vi "Register gRPC Methods.vi"(8 "error in (no error)":errorcluster, 11 "Template Server in":refnum<class "ctet_dio.lvclass">) -> (0 "error out":errorcluster, 3 "Template Server out":refnum<class "ctet_dio.lvclass">)   [LabVIEW 2019, in "ctet_dio.lvlib" / "ctet_dio.lvclass"]
uses:
  ctet_dio.lvclass
  typeDefs/Server Internal UEs.ctl
  typeDefs/Server Internal Message.ctl
  typeDefs/Server gRPC UEs.ctl
  gRPC lvSupport/Server API/typeDefs/gRPCId Cluster.ctl
  gRPC lvSupport/Server API/typeDefs/grpcId.ctl
  ctet_dio.lvclass/ctet_dio.ctl
  gRPC lvSupport/gprc-lvsupport.lvlib
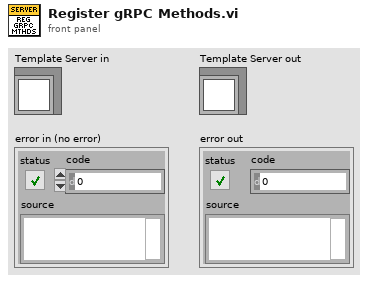
[diagram p1: front panel]
types:
  T1 = typedef "ctet_dio.lvlib/ctet_dio.lvclass/Server gRPC UEs.ctl" = cluster{"Invoke gRPC UE":refnum<user-event>, "Query gRPC UE":refnum<user-event>, "Register gRPC UE":refnum<user-event>, "OpenDISession gRPC UE":refnum<user-event>, "OpenDOSession gRPC UE":refnum<user-event>, "ReadDI gRPC UE":refnum<user-event>, "StopDI gRPC UE":refnum<user-event>, "WriteDO gRPC UE":refnum<user-event>, "CloseDISession gRPC UE":refnum<user-event>, "CloseDOSession gRPC UE":refnum<user-event>}
  T2 = typedef "ctet_dio.lvlib/ctet_dio.lvclass/Server Internal UEs.ctl" = cluster{"Invoke Internal UE":refnum<user-event>, "Query Internal UE":refnum<user-event>, "Register Internal UE":refnum<user-event>, "OpenDISession Internal UE":refnum<user-event>, "OpenDOSession Internal UE":refnum<user-event>, "ReadDI Internal UE":refnum<user-event>, "StopDI Internal UE":refnum<user-event>, "WriteDO Internal UE":refnum<user-event>, "CloseDISession Internal UE":refnum<user-event>, "CloseDOSession Internal UE":refnum<user-event>}
  T3 = typedef "ctet_dio.lvlib/gprc-lvsupport.lvlib/grpcId.ctl" = u64
  T4 = typedef "ctet_dio.lvlib/ctet_dio.lvclass/Server Internal Message UE.ctl" = refnum<user-event>
  T5 = typedef "ctet_dio.lvlib/gprc-lvsupport.lvlib/gRPCId Cluster UE.ctl" = refnum<user-event>
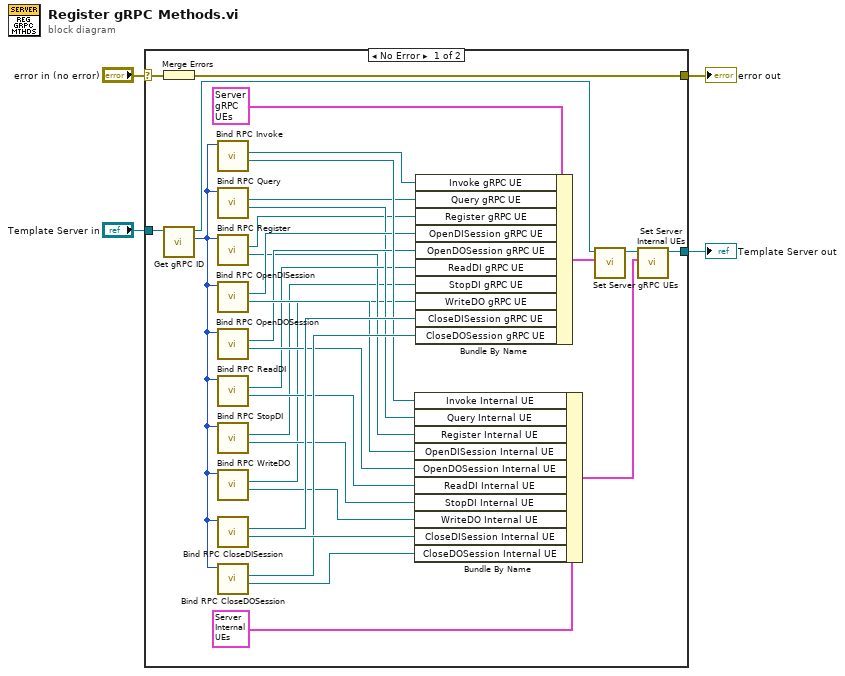
[diagram p0: block diagram]
diagram:
  n1 = case shown="No Error" "error in (no error)" {
    selector: "error in (no error)" -> [w26 w36]
    tunnel: "Template Server in" -> [w34 w37]
    tunnel: [w33 w36] -> w3
    tunnel: [w32 w37] -> w2
    frame No Error {
      n2 = Merge Errors(w26) -> (w33:errorcluster)
      n3 = call "Get gRPC ID.vi"("OOP Server in"=w34) -> ("gRPC ID"=w25:T3, "OOP Server out"=w35:refnum<class "ctet_dio.lvclass">)  [unwired: 9 in]
      n4 = call "Bind RPC Invoke.vi"("gRPCid server in"=w25) -> ("Invoke Internal UE"=w20:T4, "Invoke gRPC UE"=w19:T5)  [unwired: 7 in, 2 out]
      n5 = call "Bind RPC Query.vi"("gRPCid server in"=w25) -> ("Query Internal UE"=w14:T4, "Query gRPC UE"=w13:T5)  [unwired: 7 in, 2 out]
      n6 = call "Bind RPC Register.vi"("gRPCid server in"=w25) -> ("Register Internal UE"=w10:T4, "Register gRPC UE"=w9:T5)  [unwired: 7 in, 2 out]
      n7 = call "Bind RPC OpenDISession.vi"("gRPCid server in"=w25) -> ("OpenDISession Internal UE"=w18:T4, "OpenDISession gRPC UE"=w17:T5)  [unwired: 7 in, 2 out]
      n8 = call "Bind RPC OpenDOSession.vi"("gRPCid server in"=w25) -> ("OpenDOSession Internal UE"=w16:T4, "OpenDOSession gRPC UE"=w15:T5)  [unwired: 7 in, 2 out]
      n9 = call "Bind RPC ReadDI.vi"("gRPCid server in"=w25) -> ("ReadDI Internal UE"=w12:T4, "ReadDI gRPC UE"=w11:T5)  [unwired: 7 in, 2 out]
      n10 = call "Bind RPC StopDI.vi"("gRPCid server in"=w25) -> ("StopDI Internal UE"=w8:T4, "StopDI gRPC UE"=w7:T5)  [unwired: 7 in, 2 out]
      n11 = call "Bind RPC WriteDO.vi"("gRPCid server in"=w25) -> ("WriteDO Internal UE"=w6:T4, "WriteDO gRPC UE"=w5:T5)  [unwired: 7 in, 2 out]
      n12 = call "Bind RPC CloseDISession.vi"("gRPCid server in"=w25) -> ("CloseDISession Internal UE"=w24:T4, "CloseDISession gRPC UE"=w23:T5)  [unwired: 7 in, 2 out]
      n13 = call "Bind RPC CloseDOSession.vi"("gRPCid server in"=w25) -> ("CloseDOSession Internal UE"=w22:T4, "CloseDOSession gRPC UE"=w21:T5)  [unwired: 7 in, 2 out]
      n14 = Bundle By Name ("Bundle Internal UEs")(cluster=T2 {"Invoke Internal UE"=refnum, "Query Internal UE"=refnum, "Register Internal UE"=refnum, "OpenDISession Internal UE"=refnum, "OpenDOSession Internal UE"=refnum, "ReadDI Internal UE"=refnum, "StopDI Internal UE"=refnum, "WriteDO Internal UE"=refnum, "CloseDISession Internal UE"=refnum, "CloseDOSession Internal UE"=refnum} ("Server Internal UEs"), "Invoke Internal UE"=w20, "Query Internal UE"=w14, "Register Internal UE"=w10, "OpenDISession Internal UE"=w18, "OpenDOSession Internal UE"=w16, "ReadDI Internal UE"=w12, "StopDI Internal UE"=w8, "WriteDO Internal UE"=w6, "CloseDISession Internal UE"=w24, "CloseDOSession Internal UE"=w22) -> (w31:T2)
      n15 = Bundle By Name ("Bundle gRPC UEs")(cluster=T1 {"Invoke gRPC UE"=refnum, "Query gRPC UE"=refnum, "Register gRPC UE"=refnum, "OpenDISession gRPC UE"=refnum, "OpenDOSession gRPC UE"=refnum, "ReadDI gRPC UE"=refnum, "StopDI gRPC UE"=refnum, "WriteDO gRPC UE"=refnum, "CloseDISession gRPC UE"=refnum, "CloseDOSession gRPC UE"=refnum} ("gRPC Server Method Events"), "Invoke gRPC UE"=w19, "Query gRPC UE"=w13, "Register gRPC UE"=w9, "OpenDISession gRPC UE"=w17, "OpenDOSession gRPC UE"=w15, "ReadDI gRPC UE"=w11, "StopDI gRPC UE"=w7, "WriteDO gRPC UE"=w5, "CloseDISession gRPC UE"=w23, "CloseDOSession gRPC UE"=w21) -> (w28:T1)
      n16 = call "Set Server gRPC UEs.vi"("Server gRPC UEs"=w28, "OOP Server in"=w35) -> ("OOP Server out"=w29:refnum<class "ctet_dio.lvclass">)  [unwired: 9 in]
      n17 = call "Set Server Internal UEs.vi"("Server Internal UEs"=w31, "OOP Server in"=w29) -> ("OOP Server out"=w32:refnum<class "ctet_dio.lvclass">)  [unwired: 9 in]
    }
    frame Error {
    }
  }
  "error out" <- w3
  "Template Server out" <- w2
